vi "LaunchMonochromator.vi"(8 "error in (no error)":errorcluster) -> (0 "error out":errorcluster)   [LabVIEW 2021]
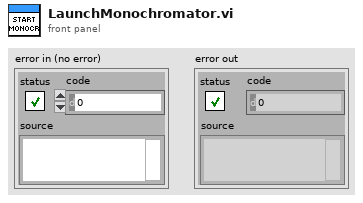
[diagram p1: front panel]
types:
  T1 = enum32{"Bad", "Idle", "Run top level", "Running"}
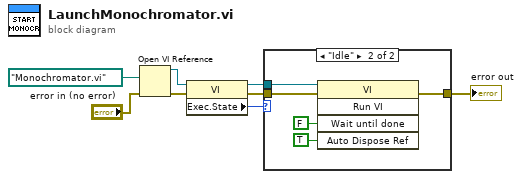
[diagram p0: block diagram]
diagram:
  n1 = Open VI Reference(vi path=path "Monochromator.vi", error in (no error)="error in (no error)") -> (vi reference=w1:refnum<vi>, error out=w4:errorcluster)  [unwired: 4 in]
  n2 = property class="VI"(reference=w1, error in=w4) -> (reference out=w5:refnum<vi>, error out=w3:errorcluster, "Exec.State"=w2:T1)
  n3 = case shown="\"Idle\"" w2 {
    tunnel: [w9 w12] -> w6
    tunnel: w5 -> [_ w11]
    tunnel: w3 -> [w9 w10]
    frame "Bad", Default {
    }
    frame "Idle" {
      n4 = invoke class="VI" method="Run VI"(reference=w11, error in=w10, "Wait until done"=FALSE ("Wait Until Done"), "Auto Dispose Ref"=TRUE ("Auto Dispose Reference")) -> (error out=w12:errorcluster)  [unwired: 1 in, 4 out]
    }
  }
  "error out" <- w6
